vi "TSCAN_Connect.vi"(8 "错误输入（无错误）":errorcluster, 11 "路径输入":path) -> (0 "错误输出":errorcluster, 3 "路径输出":path, 4 "Connect_TSCAN_Successfully":bool)   [LabVIEW 2019]
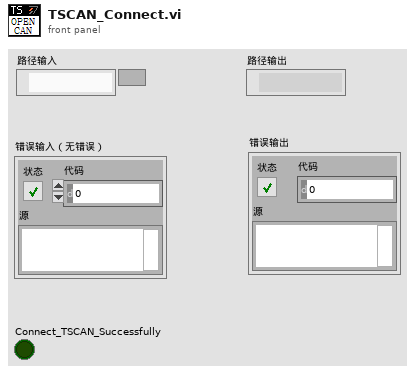
[diagram p1: front panel]
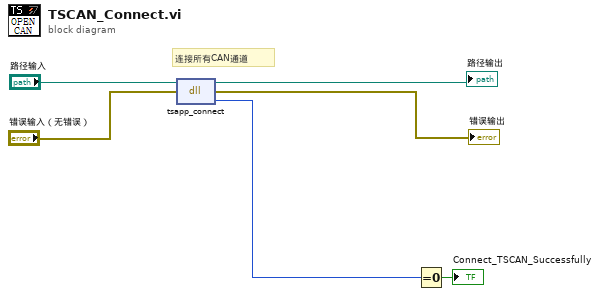
[diagram p0: block diagram]
diagram:
  # "连接所有CAN通道"
  n1 = dll-call lib="PTH2Habs CUsers\nAdministratorDesktopTS_Can通讯PathTSMaster.dll" fn="tsapp_connect"(path in="路径输入", error in="错误输入（无错误）") -> (path out=→"路径输出":path, error out=→"错误输出":errorcluster, "tsapp_connect"=w5:i32)  [unwired: 1 in]
  n2 = Equal To 0?(x=w5) -> (x = 0?=→"Connect_TSCAN_Successfully":bool)
